vi "Read Differential Pressure.vi"(8 "error in (no error)":errorcluster, 11 "VISA resource name":refnum<visa-resource-name>) -> (0 "error out":errorcluster, 2 "Differential Pressure":dbl, 3 "VISA resource name out":refnum<visa-resource-name>)   [LabVIEW 2023, in "Fluke Molbox 1 Plus.lvlib"]
doc: "Read the differential pressure value used by molbox1+ to calculate flow. The molbox1+ has upstream and downstream absolute RPTs. The pressure returned by this command is the differential pressure value that is being used by molbox1+ to calculate flow. This is the tare adjusted difference between the 2 absolute RPTs. The first 3 characters of the reply from molbox1+ make up the Ready/Not Ready condition. The differential pressure string follows it."
uses:
  Fluke Molbox 1 Plus.lvlib
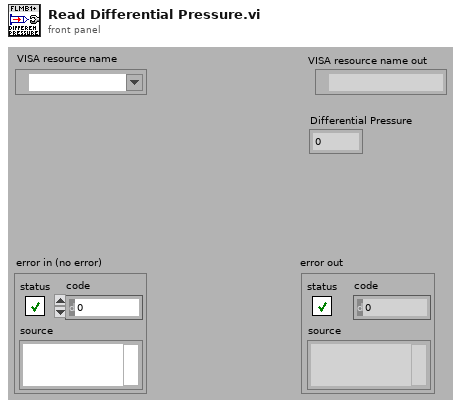
[diagram p1: front panel]
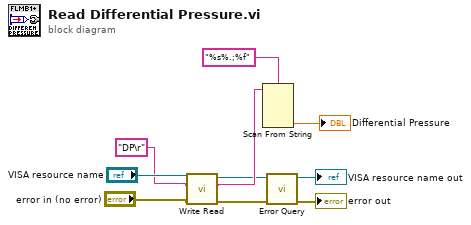
[diagram p0: block diagram]
diagram:
  n1 = call "Write Read.vi"("error in (no error)"="error in (no error)", "Write String"="DP\r" ("write buffer"), "VISA resource name"="VISA resource name") -> ("error out"=w2:errorcluster, "Read Response"=w5:string, "VISA resource name out"=w1:refnum<visa-resource-name>)  [unwired: 6 in]
  n2 = Scan From String(format string="%s%.;%f", input string=w5) -> (output 2=→"Differential Pressure":dbl)  [unwired: 5 in, 3 out]
  n3 = call "Error Query.vi"("error in (no error)"=w2, "VISA resource name"=w1) -> ("error out"=→"error out":errorcluster, "VISA resource name out"=→"VISA resource name out":refnum<visa-resource-name>)  [unwired: 6 in, 2 out]
